vi "ControlShooter.vi"(1 "State":T2) -> (0 "To Shooter\nSolenoid Loop":T1=enum."Forward")   [LabVIEW 2013]
uses:
  typedefs/subStates.ctl
  <vilib>/Rock Robotics/WPI/Solenoid/WPI_SolenoidValue.ctl
  typedefs/fg_typedef.ctl
  <vilib>/Rock Robotics/WPI/Solenoid/WPI_SolenoidGetEnum.vi
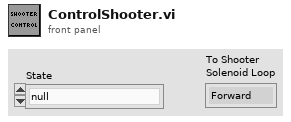
[diagram p1: front panel]
types:
  T1 = typedef "WPI_SolenoidValue.ctl" = enum16{"Off", "On", "Forward", "Reverse"}
  T2 = typedef "subStates.ctl" = enum16{"null", "wait", "driver control", "auto", "manual override", "hold position", "rotate", "pickup", "pass", "load", "goto shoot", "shoot", "end"}
  T3 = typedef "fg_typedef.ctl" = enum16{"Get", "Set"}
  T4 = typedef "WPI_DigitalInputDevRef.ctl" = cluster{"DevStatus":errorcluster, "DIO Channel":T5, "Digital Module":T6}
  T5 = typedef "FPGA_DIOChannel.ctl" = enum8{"DIO 1", "DIO 2", "DIO 3", "DIO 4", "DIO 5", "DIO 6", "DIO 7", "DIO 8", "DIO 9", "DIO 10", "DIO 11", "DIO 12", "DIO 13", "DIO 14", "Invalid"}
  T6 = typedef "FPGA_TypedefDigitalModule.ctl" = enum16{"Digital Module 1", "Digital Module 2"}
  T7 = typedef "WPI_SolenoidDevRef.ctl" = cluster{"DevStatus":errorcluster, "Solenoid Module":T8, "Forward Solenoid Channel":T9, "Reverse Solenoid Channel":T9}
  T8 = typedef "FPGA_TypedefSolenoidModule.ctl" = enum16{"Solenoid Module 1", "Solenoid Module 2"}
  T9 = typedef "WPI_SolenoidChannel.ctl" = enum8{"Solenoid 1", "Solenoid 2", "Solenoid 3", "Solenoid 4", "Solenoid 5", "Solenoid 6", "Solenoid 7", "Solenoid 8", "Invalid"}
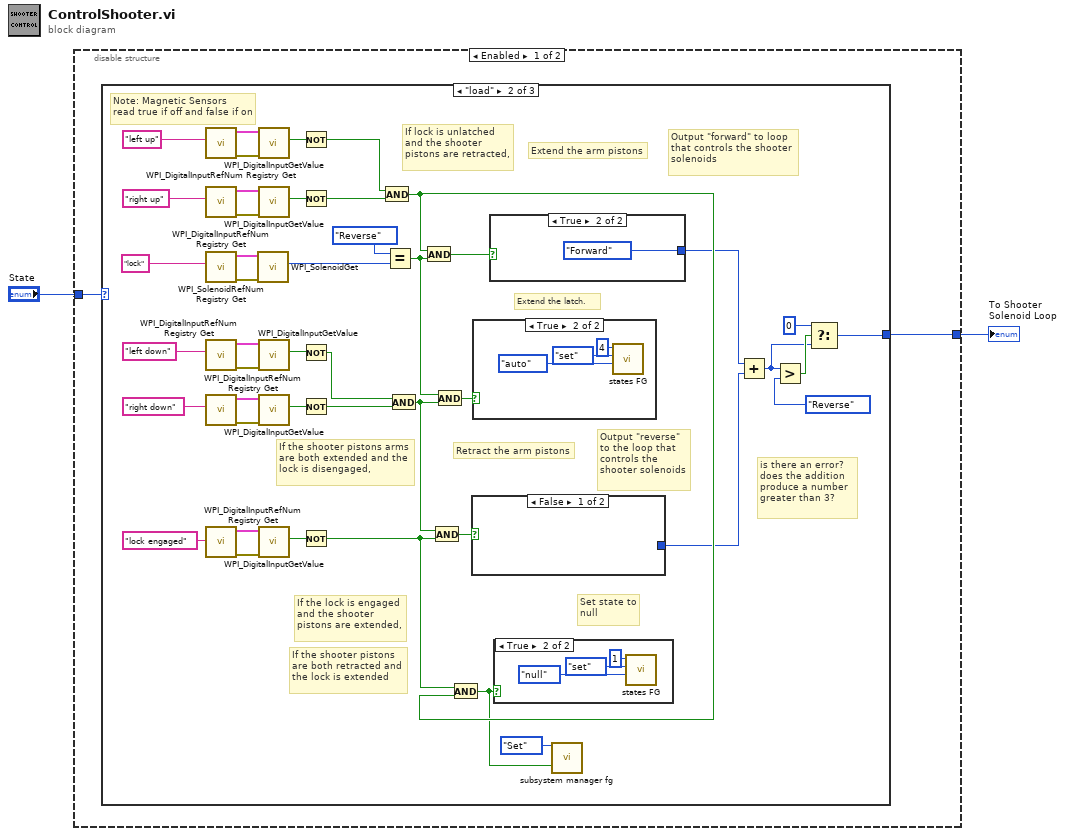
[diagram p0: block diagram]
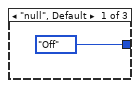
[diagram p2: hidden frame]
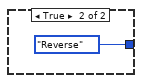
[diagram p4: hidden frame]
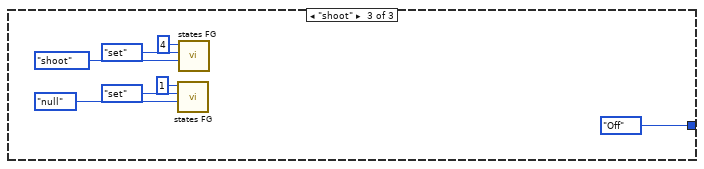
[diagram p7: hidden frame]
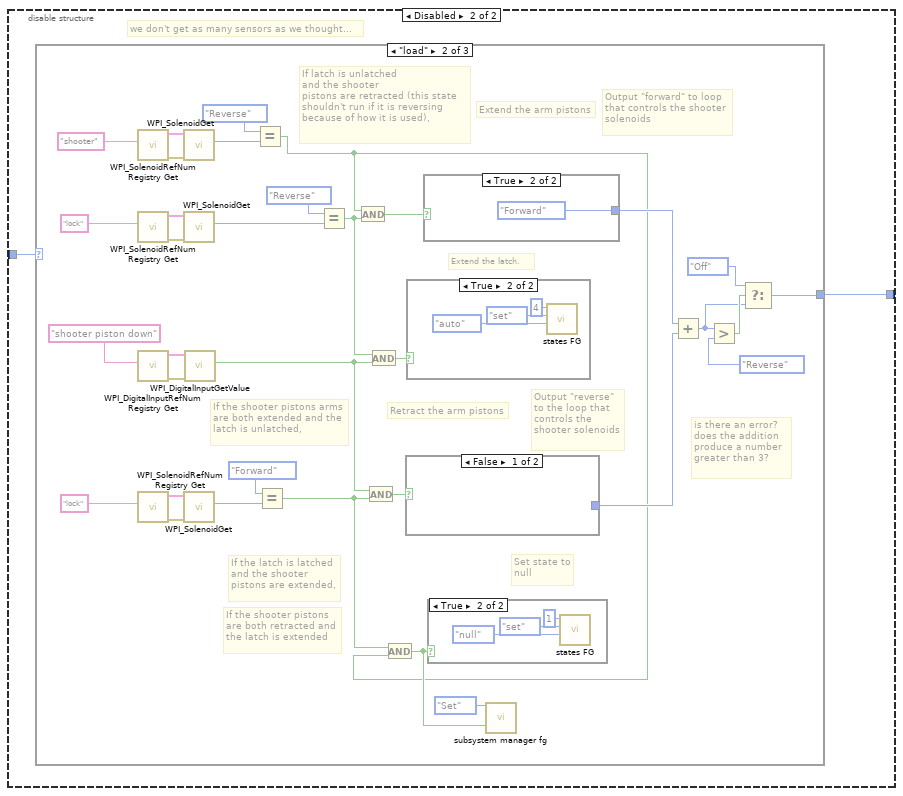
[diagram p8: hidden frame]
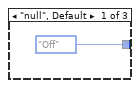
[diagram p9: hidden frame]
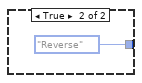
[diagram p11: hidden frame]
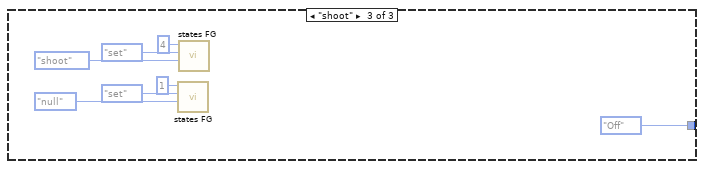
[diagram p14: hidden frame]
diagram:
  n1 = disable-structure shown="Enabled" {
    disable-tunnel: "State" -> [w4 w67]
    disable-tunnel: [w3 w66] -> w1
    frame Enabled {
      n2 = case shown="\"load\"" w4 {
        tunnel: [WPI_SolenoidValue."Off" ("To Shooter\nSolenoid Loop") w22 WPI_SolenoidValue."Off" ("To Shooter\nSolenoid Loop")] -> w3
        frame "null", Default {
        }
        frame "load" {
          # "Note: Magnetic Sensors\nread true if off and false if on"
          # "is there an error?\ndoes the addition\nproduce a number \ngreater than 3?"
          # "Output \"reverse\"\nto the loop that\ncontrols the\nshooter solenoids"
          # "Output \"forward\" to loop\nthat controls the shooter\nsolenoids"
          # "Set state to\nnull"
          # "If the shooter pistons\nare both retracted and\nthe lock is extended"
          # "If the lock is engaged\nand the shooter\npistons are extended,"
          # "Retract the arm pistons"
          # "If lock is unlatched\nand the shooter\npistons are retracted,"
          # "Extend the latch."
          # "If the shooter pistons arms\nare both extended and the\nlock is disengaged,"
          # "Extend the arm pistons"
          n3 = call <vilib>:"WPI_DigitalInputRefNum Registry Get.vi"("refnum name"="left up") -> ("error out"=w41:errorcluster, "DigitalInputDevRef"=w42:T4)  [unwired: 9 in]
          n4 = call <vilib>:"WPI_DigitalInputRefNum Registry Get.vi"("refnum name"="right up") -> ("error out"=w44:errorcluster, "DigitalInputDevRef"=w45:T4)  [unwired: 9 in]
          n5 = call <vilib>:"WPI_SolenoidRefNum Registry Get.vi"("refnum name"="lock") -> ("error out"=w50:errorcluster, "SolenoidDevRef"=w49:T7)  [unwired: 9 in]
          n6 = call <vilib>:"WPI_DigitalInputRefNum Registry Get.vi"("refnum name"="left down") -> ("error out"=w36:errorcluster, "DigitalInputDevRef"=w37:T4)  [unwired: 9 in]
          n7 = call <vilib>:"WPI_DigitalInputRefNum Registry Get.vi"("refnum name"="right down") -> ("error out"=w33:errorcluster, "DigitalInputDevRef"=w34:T4)  [unwired: 9 in]
          n8 = call <vilib>:"WPI_DigitalInputRefNum Registry Get.vi"("refnum name"="lock engaged") -> ("error out"=w16:errorcluster, "DigitalInputDevRef"=w17:T4)  [unwired: 9 in]
          n9 = call-poly <vilib>:"WPI_SolenoidGet.vi"("error in (no error)"=w50, "SolenoidDevRef"=w49) -> ("Value"=w47:T1)  [unwired: 7 in, 2 out]
          n10 = call <vilib>:"WPI_DigitalInputGetValue.vi"("error in (no error)"=w41, "DigitalInputDevRef"=w42) -> ("Value"=w7:bool)  [unwired: 7 in, 2 out]
          n11 = call <vilib>:"WPI_DigitalInputGetValue.vi"("error in (no error)"=w44, "DigitalInputDevRef"=w45) -> ("Value"=w9:bool)  [unwired: 7 in, 2 out]
          n12 = call <vilib>:"WPI_DigitalInputGetValue.vi"("error in (no error)"=w36, "DigitalInputDevRef"=w37) -> ("Value"=w11:bool)  [unwired: 7 in, 2 out]
          n13 = call <vilib>:"WPI_DigitalInputGetValue.vi"("error in (no error)"=w33, "DigitalInputDevRef"=w34) -> ("Value"=w13:bool)  [unwired: 7 in, 2 out]
          n14 = call <vilib>:"WPI_DigitalInputGetValue.vi"("error in (no error)"=w16, "DigitalInputDevRef"=w17) -> ("Value"=w15:bool)  [unwired: 7 in, 2 out]
          n15 = Not(x=w7) -> (.not. x?=w6:bool)
          n16 = Not(x=w9) -> (.not. x?=w8:bool)
          n17 = Not(x=w11) -> (.not. x?=w10:bool)
          n18 = Not(x=w13) -> (.not. x?=w12:bool)
          n19 = Not(x=w15) -> (.not. x?=w14:bool)
          n20 = And(x=w6, y=w8) -> (x .and. y?=w28:bool)
          n21 = Equal?(x=WPI_SolenoidValue."Reverse", y=w47) -> (x = y?=w29:bool)
          n22 = And(x=w10, y=w12) -> (x .and. y?=w30:bool)
          n23 = And(x=w28, y=w29) -> (x .and. y?=w39:bool)
          n24 = And(x=w30, y=w14) -> (x .and. y?=w31:bool)
          n25 = And(x=w29, y=w30) -> (x .and. y?=w38:bool)
          n26 = And(x=w14, y=w28) -> (x .and. y?=w19:bool)
          n27 = case shown="False" w31 {
            tunnel: [_ WPI_SolenoidValue."Reverse" ("Value")] -> w21
            frame False {
            }
            frame True {
            }
          }
          n28 = case shown="True" w38 {
            frame False {
            }
            frame True {
              n29 = call "states FG.vi"("subState in"=subStates."auto", "menu (get)"=enum16{"set", "get"}."set", "Loop ID"=4) -> ()  [unwired: 5 in, 4 out]
            }
          }
          n30 = case shown="True" w39 {
            tunnel: [_ WPI_SolenoidValue."Forward" ("Value")] -> w27
            frame False {
            }
            frame True {
            }
          }
          n31 = case shown="True" w19 {
            frame False {
            }
            frame True {
              n32 = call "states FG.vi"("subState in"=subStates."null", "menu (get)"=enum16{"set", "get"}."set", "Loop ID"=1) -> ()  [unwired: 5 in, 4 out]
            }
          }
          n33 = call "subsystem manager fg.vi"("Menu"=fg_typedef."Set", "Shooter Cocked"=w19) -> ()  [unwired: 13 in, 5 out]
          n34 = Add(x=w27, y=w21) -> (x+y=w24:u16)
          n35 = Greater?(x=w24, y=WPI_SolenoidValue."Reverse" ("Value")) -> (0:w25:bool)
          n36 = Select(t=0, s=w25, f=w24) -> (s? t:f=w22:i32)
        }
        frame "shoot" {
          n37 = call "states FG.vi"("subState in"=subStates."null", "menu (get)"=enum16{"set", "get"}."set", "Loop ID"=1) -> ()  [unwired: 5 in, 4 out]
          n38 = call "states FG.vi"("subState in"=subStates."shoot", "menu (get)"=enum16{"set", "get"}."set", "Loop ID"=4) -> ()  [unwired: 5 in, 4 out]
        }
      }
    }
    frame Disabled {
      # "we don't get as many sensors as we thought..."
      n39 = case shown="\"load\"" w67 {
        tunnel: [WPI_SolenoidValue."Off" ("To Shooter\nSolenoid Loop") w80 WPI_SolenoidValue."Off" ("To Shooter\nSolenoid Loop")] -> w66
        frame "null", Default {
        }
        frame "load" {
          # "is there an error?\ndoes the addition\nproduce a number \ngreater than 3?"
          # "Output \"reverse\"\nto the loop that\ncontrols the\nshooter solenoids"
          # "Output \"forward\" to loop\nthat controls the shooter\nsolenoids"
          # "Set state to\nnull"
          # "If the shooter pistons\nare both retracted and\nthe latch is extended"
          # "If the latch is latched\nand the shooter\npistons are extended,"
          # "Retract the arm pistons"
          # "If latch is unlatched\nand the shooter\npistons are retracted (this state shouldn't run if it is reversing because of how it is used),"
          # "Extend the latch."
          # "If the shooter pistons arms\nare both extended and the\nlatch is unlatched,"
          # "Extend the arm pistons"
          n40 = call <vilib>:"WPI_SolenoidRefNum Registry Get.vi"("refnum name"="shooter") -> ("error out"=w72:errorcluster, "SolenoidDevRef"=w73:T7)  [unwired: 9 in]
          n41 = call <vilib>:"WPI_SolenoidRefNum Registry Get.vi"("refnum name"="lock") -> ("error out"=w102:errorcluster, "SolenoidDevRef"=w101:T7)  [unwired: 9 in]
          n42 = call <vilib>:"WPI_DigitalInputRefNum Registry Get.vi"("refnum name"="shooter piston down") -> ("error out"=w94:errorcluster, "DigitalInputDevRef"=w95:T4)  [unwired: 9 in]
          n43 = call <vilib>:"WPI_SolenoidRefNum Registry Get.vi"("refnum name"="lock") -> ("error out"=w92:errorcluster, "SolenoidDevRef"=w91:T7)  [unwired: 9 in]
          n44 = call-poly <vilib>:"WPI_SolenoidGet.vi"("error in (no error)"=w72, "SolenoidDevRef"=w73) -> ("Value"=w74:T1)  [unwired: 7 in, 2 out]
          n45 = call-poly <vilib>:"WPI_SolenoidGet.vi"("error in (no error)"=w102, "SolenoidDevRef"=w101) -> ("Value"=w99:T1)  [unwired: 7 in, 2 out]
          n46 = call-poly <vilib>:"WPI_SolenoidGet.vi"("error in (no error)"=w92, "SolenoidDevRef"=w91) -> ("Value"=w89:T1)  [unwired: 7 in, 2 out]
          n47 = call <vilib>:"WPI_DigitalInputGetValue.vi"("error in (no error)"=w94, "DigitalInputDevRef"=w95) -> ("Value"=w76:bool)  [unwired: 7 in, 2 out]
          n48 = Equal?(x=WPI_SolenoidValue."Reverse", y=w74) -> (x = y?=w70:bool)
          n49 = Equal?(x=WPI_SolenoidValue."Forward", y=w89) -> (x = y?=w85:bool)
          n50 = Equal?(x=WPI_SolenoidValue."Reverse", y=w99) -> (x = y?=w86:bool)
          n51 = And(x=w70, y=w86) -> (x .and. y?=w97:bool)
          n52 = And(x=w76, y=w85) -> (x .and. y?=w87:bool)
          n53 = And(x=w86, y=w76) -> (x .and. y?=w96:bool)
          n54 = And(x=w85, y=w70) -> (x .and. y?=w77:bool)
          n55 = case shown="False" w87 {
            tunnel: [_ WPI_SolenoidValue."Reverse" ("Value")] -> w79
            frame False {
            }
            frame True {
            }
          }
          n56 = case shown="True" w96 {
            frame False {
            }
            frame True {
              n57 = call "states FG.vi"("subState in"=subStates."auto", "menu (get)"=enum16{"set", "get"}."set", "Loop ID"=4) -> ()  [unwired: 5 in, 4 out]
            }
          }
          n58 = case shown="True" w97 {
            tunnel: [_ WPI_SolenoidValue."Forward" ("Value")] -> w84
            frame False {
            }
            frame True {
            }
          }
          n59 = case shown="True" w77 {
            frame False {
            }
            frame True {
              n60 = call "states FG.vi"("subState in"=subStates."null", "menu (get)"=enum16{"set", "get"}."set", "Loop ID"=1) -> ()  [unwired: 5 in, 4 out]
            }
          }
          n61 = call "subsystem manager fg.vi"("Menu"=fg_typedef."Set", "Shooter Cocked"=w77) -> ()  [unwired: 13 in, 5 out]
          n62 = Add(x=w84, y=w79) -> (x+y=w81:u16)
          n63 = Greater?(x=w81, y=WPI_SolenoidValue."Reverse" ("Value")) -> (0:w82:bool)
          n64 = Select(t=WPI_SolenoidValue."Off" ("Value"), s=w82, f=w81) -> (s? t:f=w80:u16)
        }
        frame "shoot" {
          n65 = call "states FG.vi"("subState in"=subStates."null", "menu (get)"=enum16{"set", "get"}."set", "Loop ID"=1) -> ()  [unwired: 5 in, 4 out]
          n66 = call "states FG.vi"("subState in"=subStates."shoot", "menu (get)"=enum16{"set", "get"}."set", "Loop ID"=4) -> ()  [unwired: 5 in, 4 out]
        }
      }
    }
  }
  "To Shooter\nSolenoid Loop" <- w1
